vi "Draw Dot.vi"(6 "Coords":T1, 8 "error in (no error)":errorcluster, 9 "Data In":T2, 11 "Waveform Ref":refnum<vi>) -> (0 "error out":errorcluster, 1 "Plot Number":i32, 3 "XY Strings":cluster{"X":string, "Y":string})   [LabVIEW 2013, in "XGrapher.xctl"]
uses:
  XGrapher.xctl
  Data 1.ctl
  Typedefs/Xctrl-Data array.ctl
  Typedefs/Xcrtl-Data format definition.ctl
  Typedefs/Xctl-XY data type definition.ctl
  Typedefs/Xctrl-ROI type enum.ctl
  <vilib>/Utility/miscctls.llb/LVPoint32TypeDef.ctl
panel:
  out "size(s)":i32[](array[numeric])
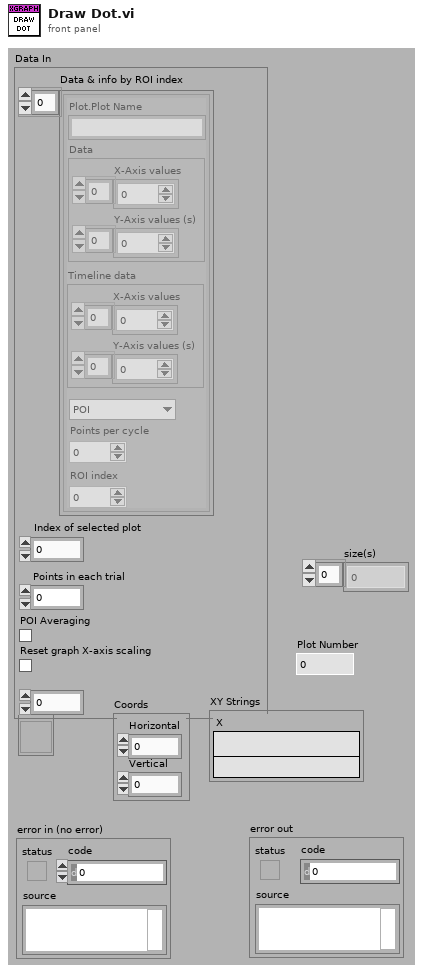
[diagram p1: front panel]
types:
  T1 = typedef "LVPoint32TypeDef.ctl" = cluster{"Horizontal":i32, "Vertical":i32}
  T2 = typedef "XGrapher.xctl/Data 1.ctl" = cluster{"Data & info by ROI index":T3, "Index of selected plot":u16, "Points in each trial":i32, "POI Averaging":bool, "Reset graph X-axis scaling":bool, "Selected point index in MSCN (unity based)":u16}
  T3 = typedef "Xctrl-Data array.ctl" = T4[]
  T4 = typedef "XGrapher.xctl/Xcrtl-Data format definition.ctl" = cluster{"Plot.Plot Name":string, "Data":T5, "Timeline data":T5, "Type":T6, "Points per cycle":u16, "ROI index":u16}
  T5 = typedef "XGrapher.xctl/Xctl-XY data type definition.ctl" = cluster{"X-Axis values":sgl[], "Y-Axis values (s)":i32[]}
  T6 = typedef "Xctrl-ROI type enum.ctl" = enum16{"POI", "Mini-scan", "Group"}
  T7 = cluster{"Width":u16, "Style":enum32{"Solid", "Dash", "Dot", "DashDot", "DashDotDot"}}
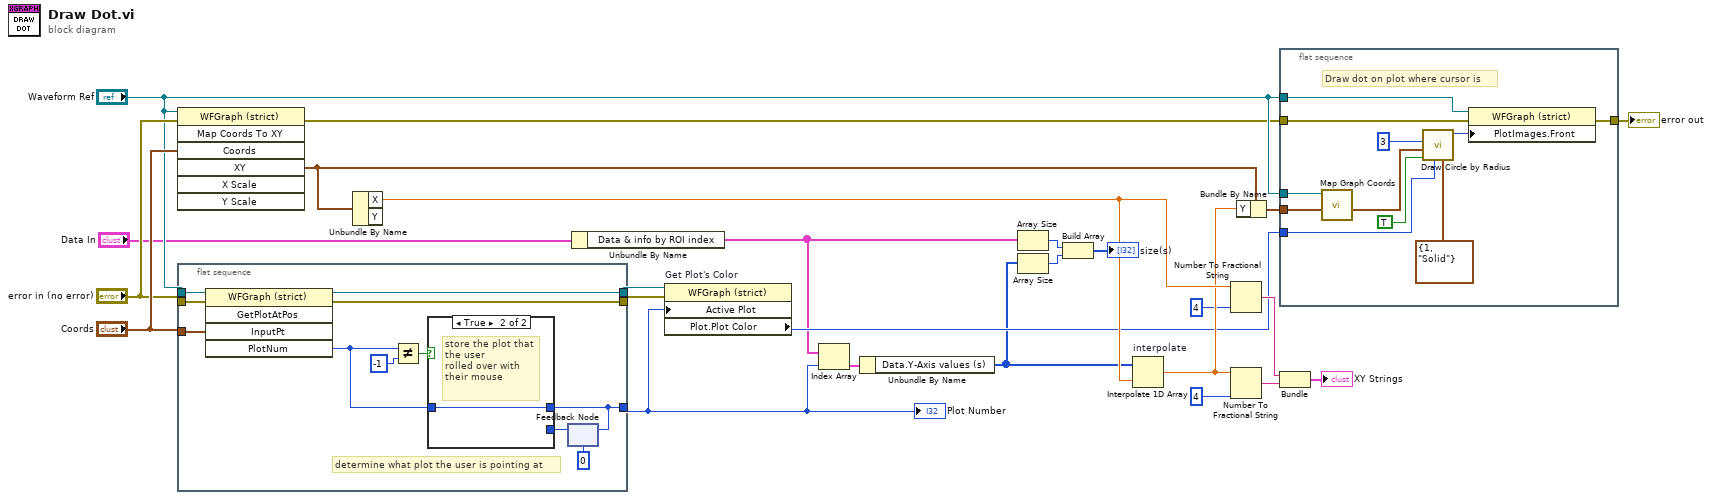
[diagram p0: block diagram]
diagram:
  n1 = invoke on="Invoke Node" class="WFGraph (strict)" method="Map Coords To XY"(reference="Waveform Ref", error in="error in (no error)", "Coords"="Coords") -> (error out=w14:errorcluster, "XY"=w24:cluster{"X":dbl, "Y":dbl})  [unwired: 4 in, 5 out]
  n2 = flat-sequence {
    tunnel: "Coords" -> [w36]
    tunnel: "error in (no error)" -> [w35]
    tunnel: [w29] -> w9
    tunnel: [w28] -> w18
    tunnel: [w27] -> w17
    tunnel: "Waveform Ref" -> [w26]
    frame #0 {
      # "determine what plot the user is pointing at"
      n3 = invoke on="Invoke Node" class="WFGraph (strict)" method="GetPlotAtPos"(reference=w26, error in=w35, "InputPt"=w36) -> (reference out=w27:refnum<vi>, error out=w28:errorcluster, "PlotNum"=w32:i32)  [unwired: 2 in, 2 out]
      n4 = Not Equal?(x=w32, y=-1) -> (x != y?=w33:bool)
      n5 = feedback #1(0 ("PlotNum")) -> (w31:i32)
      n6 = case shown="True" w33 {
        tunnel: [w37 w38] -> w29
        tunnel: w32 -> [_ w38]
        tunnel: w31 -> [w37 _]
        frame False {
        }
        frame True {
          # "store the plot that the user\nrolled over with their mouse"
        }
      }
      n7 = feedback-in #1(w29) -> ()
    }
  }
  n8 = Unbundle By Name(w24) -> ("X"=w13:dbl)  [unwired: 1 out]
  n9 = Unbundle By Name("Data In") -> ("Data & info by ROI index"=w5:T3)
  n10 = property on="Get Plot's Color" class="WFGraph (strict)"(reference=w17, error in=w18, "Active Plot"=w9) -> ("Plot.Plot Color"=w8:u32)  [unwired: 2 out]
  n11 = Index Array(array=w5, index=w9) -> (element=w6:T4)
  n12 = Unbundle By Name(w6) -> ("Data.Y-Axis values (s)"=w4:i32[])
  n13 = Array Size(array=w5) -> (size(s)=w3:i32)
  n14 = Array Size(array=w4) -> (size(s)=w2:i32)
  n15 = Build Array(w3, w2) -> (→"size(s)":i32[])
  n16 = Interpolate 1D Array "interpolate"(1:w13, 2:w4) -> (0:w12:dbl)
  n17 = Number To Fractional String(number=w13, precision (6)=i16 4) -> (F-format string=w21:string)  [unwired: 2 in]
  n18 = Number To Fractional String(number=w12, precision (6)=i16 4) -> (F-format string=w20:string)  [unwired: 2 in]
  n19 = Bundle By Name(cluster=w24, "Y"=w12) -> (w25:cluster{"X":dbl, "Y":dbl})
  n20 = flat-sequence {
    tunnel: w25 -> [w49]
    tunnel: w8 -> [w44]
    tunnel: "Waveform Ref" -> [w43]
    tunnel: "Waveform Ref" -> [w41]
    tunnel: [w40] -> w15
    tunnel: w14 -> [w39]
    frame #0 {
      # "Draw dot on plot where cursor is"
      n21 = call "Map Graph Coords.vi"("XY"=w49, "Timeline Graph in"=w43) -> ("Coords"=w47:cluster{i32, i32})  [unwired: 8 in, 1 out]
      n22 = call <vilib>:"Draw Circle by Radius.vi"("pen"=T7 {"Width"=1, "Style"=enum."Solid"}, "color(black)"=w44, "fill?(F)"=TRUE, "pixel center"=w47, "radius"=i16 3) -> ("new picture"=w42:picture)  [unwired: 3 in, 3 out]
      n23 = property on="Property Node" class="WFGraph (strict)"(reference=w41, error in=w39, "PlotImages.Front"=w42) -> (error out=w40:errorcluster)  [unwired: 1 out]
    }
  }
  n24 = Bundle(w21, w20) -> (→"XY Strings":cluster{string, string})  [unwired: 1 in]
  "Plot Number" <- w9
  "error out" <- w15
